vi "CRC_8_CCIT.vi"(11 "Data String":string) -> (3 "Numeric":u8 format="%x")   [LabVIEW 2020]
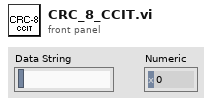
[diagram p1: front panel]
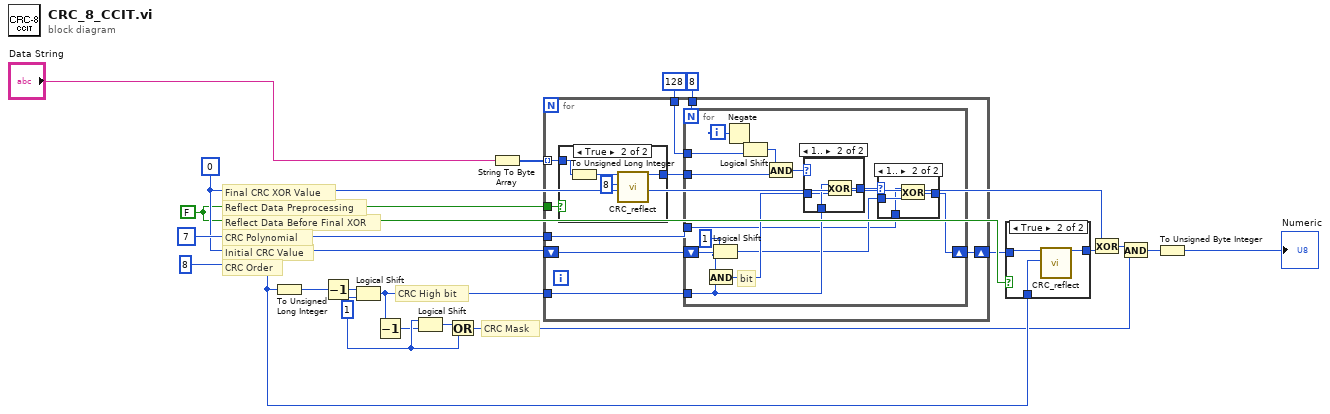
[diagram p0: block diagram]
diagram:
  w18 = u8 8 ("CRC Order")
  w15 = FALSE
  w16 = u32 0 ("Initial CRC Value")
  w5 = u32 1 ("x")
  # "CRC Order"
  # "Initial CRC Value"
  # "CRC Polynomial"
  # "Reflect Data Before Final XOR"
  # "Reflect Data Preprocessing"
  # "Final CRC XOR Value"
  # "CRC Mask"
  # "CRC High bit"
  n1 = To Unsigned Long Integer(number=w18) -> (unsigned 32bit integer=w13:u32)
  n2 = Decrement(x=w13) -> (x-1=w1:u32)
  n3 = Logical Shift(y=w1, x=w5) -> (x << y=w2:u32)
  n4 = Decrement(x=w2) -> (x-1=w3:u32)
  n5 = Logical Shift(y=w5, x=w3) -> (x << y=w4:u32)
  n6 = Or(x=w4, y=w5) -> (x .or. y?=w12:u32)
  n7 = String To Byte Array(string="Data String") -> (unsigned byte array=w20:u8[])
  n8 = for {
    shift-right: [w22] -> w9
    shift-left: w16 -> [w27]
    tunnel: w2 -> [w26]
    tunnel: w20 -> [w21] mode=indexing
    tunnel: w15 -> [w29]
    tunnel: u8 8 ("Bits") -> [w28]
    tunnel: u32 128 -> [w25]
    tunnel: u32 7 ("CRC Polynomial") -> [w23]
    n9 = case shown="True" w29 {
      tunnel: [w52 w55] -> w24
      tunnel: w21 -> [w52 w54]
      frame False {
      }
      frame True {
        n10 = To Unsigned Long Integer(number=w54) -> (unsigned 32bit integer=w53:u32)
        n11 = call "CRC_reflect.vi"("CRC"=w53, "Bits"=u8 8) -> ("Reflected CRC"=w55:u32)  [unwired: 16 in, 1 out]
      }
    }
    n12 = for {
      N: w28 -> [_]
      shift-right: [w30] -> w22
      shift-left: w27 -> [w43]
      tunnel: w26 -> [w36]
      tunnel: w25 -> [w41]
      tunnel: w24 -> [w40]
      tunnel: w23 -> [w33]
      i -> [w32]
      # "bit"
      n13 = And(x=w43, y=w36) -> (x .and. y?=w37:u32)
      n14 = Logical Shift(y=u32 1, x=w43) -> (x << y=w34:u32)
      n15 = Negate(x=w32) -> (-x=w31:i32)
      n16 = Logical Shift(y=w31, x=w41) -> (x << y=w39:u32)
      n17 = And(x=w39, y=w40) -> (x .and. y?=w38:u32)
      n18 = case shown="1.." w38 {
        tunnel: w37 -> [w48 w49]
        tunnel: [w48 w51] -> w35
        tunnel: w36 -> [_ w50]
        frame ..0 {
        }
        frame 1.. {
          n19 = Exclusive Or(1:w49, 2:w50) -> (0:w51:u32)
        }
      }
      n20 = case shown="1.." w35 {
        tunnel: w34 -> [w44 w46]
        tunnel: [w44 w47] -> w30
        tunnel: w33 -> [_ w45]
        frame ..0 {
        }
        frame 1.. {
          n21 = Exclusive Or(1:w46, 2:w45) -> (0:w47:u32)
        }
      }
    }
  }
  n22 = case shown="True" w15 {
    tunnel: w9 -> [w57 w60]
    tunnel: [w57 w59] -> w10
    tunnel: w18 -> [_ w58]
    frame False {
    }
    frame True {
      n23 = call "CRC_reflect.vi"("CRC"=w60, "Bits"=w58) -> ("Reflected CRC"=w59:u32)  [unwired: 16 in, 1 out]
    }
  }
  n24 = Exclusive Or(1:w10, 2:w16) -> (0:w11:u32)
  n25 = And(x=w11, y=w12) -> (x .and. y?=w19:u32)
  n26 = To Unsigned Byte Integer(number=w19) -> (unsigned 8bit integer=→"Numeric":u8)
